vi "shared memory write.vi"(0 "refnum in":refnum<file>, 5 "Data Array":dbl[](array[numeric]), 7 "File Array Allocation":dbl[](array[numeric]), 9 "Counter":i32, 11 "error in":errorcluster) -> (4 "refnum out":refnum<file>, 6 "Data Array Out":dbl[](array[numeric]), 8 "File Array Allocation Out":dbl[](array[numeric]), 15 "error out":errorcluster)   [LabVIEW 2013]
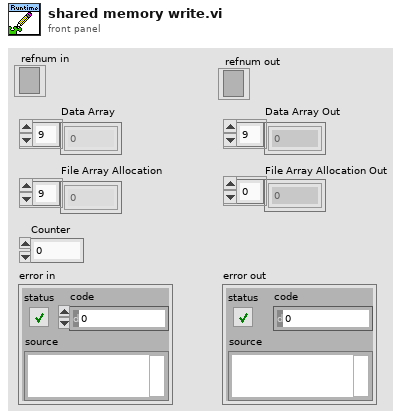
[diagram p1: front panel]
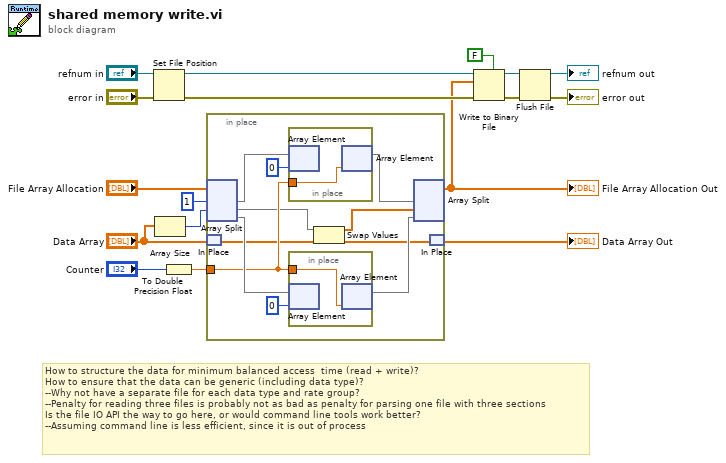
[diagram p0: block diagram]
diagram:
  # "How to structure the data for minimum balanced access  time (read + write)?\nHow to ensure that the data can be generic (including data type)?\n--Why not have a separate file for each data type and rate group?\n--Penalty for reading three files is probably not as bad as penalty for parsing one file with three sections\nIs the file IO API the way to go here, or would command line tools work better?\n--Assuming command line is less efficient, since it is out of process"
  n1 = Set File Position(refnum="refnum in", error in="error in") -> (refnum out=w14:refnum<file>, error out=w15:errorcluster)  [unwired: 2 in]
  n2 = Array Size(array="Data Array") -> (size(s)=w4:i32)
  n3 = To Double Precision Float(number="Counter") -> (double precision float=w5:dbl)
  n4 = in-place {
    in-place-border: w5 -> [w25]
    n5 = in-place-split #1("File Array Allocation", 1, w4) -> (w28:dbl[], w21:dbl[], w26:dbl[])
    n6 = in-place-match #2("Data Array") -> (w19:dbl[])
    n7 = in-place {
      in-place-border: w25 -> [w30]
      n8 = in-place-array #3(w28, 0) -> ()  [unwired: 1 out]
      n9 = in-place-array #3(w30) -> (w27:dbl[])  [unwired: 1 out]
    }
    n10 = in-place {
      in-place-border: w25 -> [w29]
      n11 = in-place-array #4(w26, 0) -> ()  [unwired: 1 out]
      n12 = in-place-array #4(w29) -> (w24:dbl[])  [unwired: 1 out]
    }
    n13 = Swap Values(12:w21, 14:w19) -> (1:w20:dbl[], 3:w18:dbl[])  [unwired: 1 in]
    n14 = in-place-split #1(w27, w20, w24) -> (w3:dbl[])  [unwired: 2 out]
    n15 = in-place-match #2(w18) -> (→"Data Array Out":dbl[])
  }
  "File Array Allocation Out" <- w3
  n16 = Write to Binary File(file (use dialog)=w14, data=w3, error in=w15, 5:FALSE ("prepend array or string size? (T)")) -> (refnum out=w12:refnum<file>, error out=w11:errorcluster)  [unwired: 2 in, 1 out]
  n17 = Flush File(refnum=w12, error in=w11) -> (refnum out=→"refnum out":refnum<file>, error out=→"error out":errorcluster)
